vi "Get DMA wrapper.vi"(7 "pDMAout":T1, 8 "error in (no error)":errorcluster caption="错误输入（无错误）", 9 "iAddr":i32, 10 "dwCanNodeId":u32, 11 "dwDevIndex":u32) -> (0 "error out":errorcluster caption="错误输出", 3 "function return":u32, 5 "pDMAout out":T1)   [LabVIEW 2016, in "UISimCanFunc_wrapper.lvlib"]
doc: "_declspec (dllexport) DWORD GetDMA_wrapper(DWORD dwDevIndex, DWORD dwCanNodeId, INT iAddr, P_DMA_OBJ pDMAout);"
uses:
  <userlib>/UISimCanFunc_wrapper/UISimCanFunc_wrapper.lvlib
  <userlib>/UISimCanFunc_wrapper/UISimCanFunc_wrapper.dll
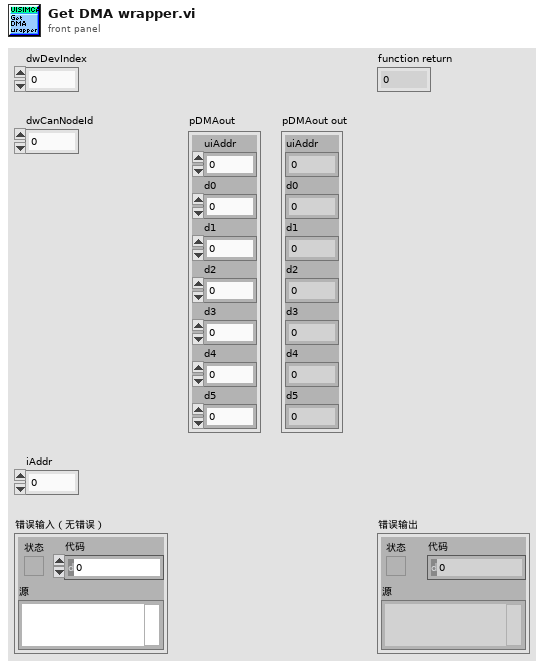
[diagram p1: front panel]
types:
  T1 = cluster{"uiAddr":u32, "d0":u8, "d1":u8, "d2":u8, "d3":u8, "d4":u8, "d5":u8}
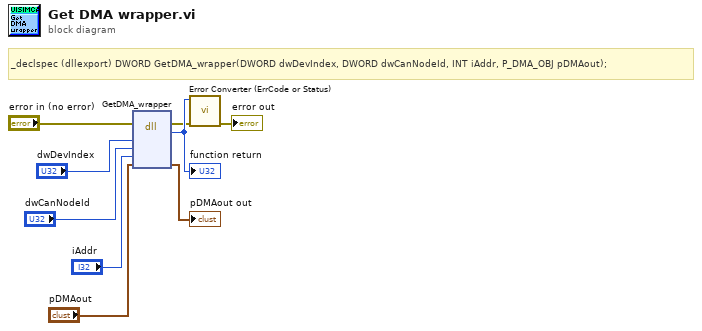
[diagram p0: block diagram]
diagram:
  # "_declspec (dllexport) DWORD GetDMA_wrapper(DWORD dwDevIndex, DWORD dwCanNodeId, INT iAddr, P_DMA_OBJ pDMAout);"
  n1 = dll-call lib="C:/Program Files (x86)/National Instruments/LabVIEW 2016/user.lib/UISimCanFunc_wrapper/UISimCanFunc_wrapper.*" fn="GetDMA_wrapper"(error in="error in (no error)", "dwDevIndex"="dwDevIndex", "dwCanNodeId"="dwCanNodeId", "iAddr"="iAddr", "pDMAout"="pDMAout") -> (error out=w2:errorcluster, w9:u32, "pDMAout"=→"pDMAout out":T1)  [unwired: 5 in, 1 out]
  "function return" <- w9
  n2 = call <userlib>:"Error Converter (ErrCode or Status).vi"("error in (no error)"=w2, "error code"=w9) -> ("error out"=→"error out":errorcluster)  [unwired: 9 in]
